vi "Fetch Raw File Data.vi"(8 "error in (no error)":errorcluster, 9 "Read File Name (\"\")":string, 11 "VISA resource name":refnum<visa-resource-name>) -> (0 "error out":errorcluster, 2 "Data":string, 3 "VISA resource name out":refnum<visa-resource-name>)   [LabVIEW 2020, in "Yokogawa GX Series.lvlib"]
doc: "This VI reads the data of internal memory and external medium(ex. CF card) and save to File for the <B>DX1000/DX2000 series</B>.\n\nSupported: \n Internal memory: *.DAD, *.DAE\n External medium: all files\nNot Supported: \n *.DAM, *.DAR(internal memory)"
uses:
  <instrlib>/Yokogawa GX Series/Yokogawa GX Series.lvlib
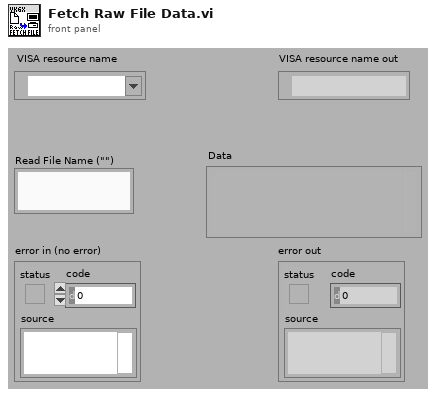
[diagram p1: front panel]
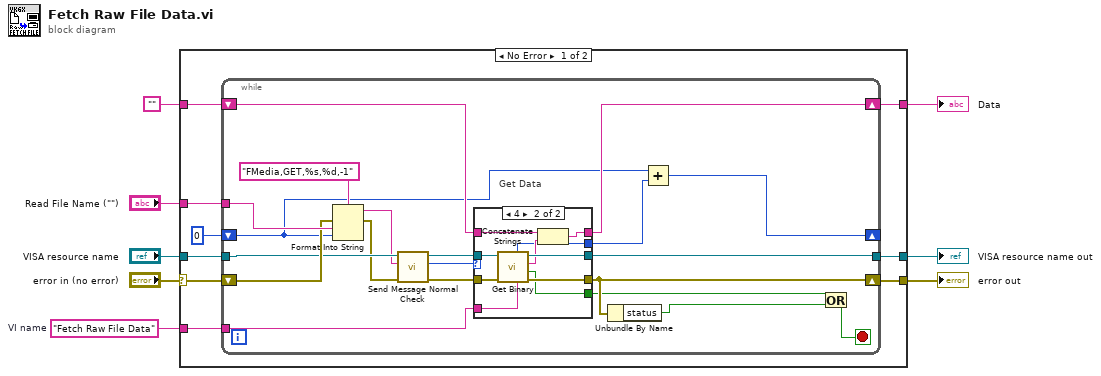
[diagram p0: block diagram]
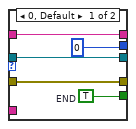
[diagram p2: hidden frame]
diagram:
  w8 = "Fetch Raw File Data"  # VI name
  n1 = case shown="No Error" "error in (no error)" {
    selector: "error in (no error)" -> [w10 w53]
    tunnel: w8 -> [w17 _]
    tunnel: "" -> [w16 w55]
    tunnel: [w15 w54] -> w6
    tunnel: [w14 w55] -> w5
    tunnel: [w13 w53] -> w4
    tunnel: "Read File Name (\"\")" -> [w12 _]
    tunnel: "VISA resource name" -> [w11 w54]
    frame No Error {
      n2 = while {
        tunnel: w17 -> [w37]
        tunnel: [w35] -> w15
        shift-right: [w34] -> w14
        shift-left: w16 -> [w36]
        shift-right: [w32] -> w13
        shift-left: w10 -> [w29]
        tunnel: w12 -> [w30]
        tunnel: w11 -> [w28]
        shift-right: [w20] -> _
        shift-left: 0 -> [w21]
        stop <- w33 stop-if-true
        # "Get Data"
        n3 = Format Into String(format string="FMedia,GET,%s,%d,-1", error in=w29, w30, w21) -> (resulting string=w26:string, error out=w27:errorcluster)  [unwired: 1 in]
        n4 = call <instrlib>:"Send Message Normal Check.vi"("error in (no error)"=w27, "Send Message (\"\")"=w26, "VISA resource name"=w28) -> ("error out"=w23:errorcluster, "Response Type"=w24:i32, "VISA resource name out"=w25:refnum<visa-resource-name>)  [unwired: 3 in, 3 out]
        n5 = case shown="4" w24 {
          tunnel: w23 -> [w41 w49]
          tunnel: w25 -> [w42 w50]
          tunnel: [w42 w46] -> w35
          tunnel: [w41 w47] -> w32
          tunnel: w36 -> [w40 w52]
          tunnel: [w40 w51] -> w34
          tunnel: [w39 w43] -> w18
          tunnel: w37 -> [_ w48]
          tunnel: [0 w44] -> w22
          frame 0, Default {
            w39 = TRUE  # END
          }
          frame 4 {
            n6 = call <instrlib>:"Get Binary.vi"("Source (\"\")"=w48, "error in (no error)"=w49, "VISA resource name"=w50) -> ("error out"=w47:errorcluster, "End of Data"=w43:bool, "Binary Data"=w45:string, "VISA resource name out"=w46:refnum<visa-resource-name>, "Read count"=w44:i32)  [unwired: 1 in, 3 out]
            n7 = Concatenate Strings(w52, w45) -> (w51:string)
          }
        }
        n8 = Unbundle By Name(w32) -> ("status"=w19:bool)
        n9 = Add(x=w21, y=w22) -> (x+y=w20:i32)
        n10 = Or(x=w18, y=w19) -> (x .or. y?=w33:bool)
      }
    }
    frame Error {
    }
  }
  "error out" <- w4
  "VISA resource name out" <- w6
  "Data" <- w5
